vi "WPI_CANTalonSRX_RequestParameter.vi"(8 "error in (no error)":errorcluster, 10 "Parameter":T1=1 items=["Slot 0 - P"=1, "Slot 0 - I"=2, "Slot 0 - D"=3, "Slot 0 - F"=4, "Slot 0 - I Zone"=5, "Slot 0 - Ramp Rate"=6, "Slot 1 - P"=11, "Slot 1 - I"=12, "Slot 1 - D"=13, "Slot 1 - F"=14, "Slot 1 - I Zone"=15, "Slot 1 - Ramp Rate"=16, "Soft Limit - Forward"=21, "Soft Limit - Reverse"=22, "Soft Limit - Forward Enable"=23, "Soft Limit - Reverse Enable"=24, "On Boot - Brake Mode"=31, "On Boot - Limit Normally Closed - Forward"=32, "On Boot - Limit Normally Closed - Reverse"=33, "On Boot - Limit Disabled - Forward"=34, "On Boot - Limit Disabled - Reverse"=35, "Fault - Over Temp"=41, "Fault - Under Voltage"=42, "Fault - Forward Limit"=43, "Fault - Reverse Limit"=44, "Fault - Hardware Failure"=45, "Fault - Forward Soft Limit"=46, "Fault - Reverse Soft Limit"=47, "Sticky Fault - Over Temp"=48, "Sticky Fault - Under Voltage"=49, "Sticky Fault - Forward Limit"=50, "Sticky Fault - Reverse Limit"=51, "Sticky Fault - Forward Soft Limit"=52, "Sticky Fault - Reverse Soft Limit"=53, "Applied Throttle"=61, "Closed-Loop Error"=62, "Select Feedback Device"=63, "Reverse Closed-Loop Output"=64, "Mode Select"=65, "Profile Slot Select"=66, "Ramp Throttle"=67, "Reverse Feedback Sensor"=68, "Limit Switch Enabled"=69, "Limit Switch Closed - Forward"=70, "Limit Switch Closed - Reverse"=71, "Sensor Position"=73, "Sensor Velocity"=74, "Current"=75, "Brake is Enabled"=76, "Encoder Position"=77, "Encoder Velocity"=78, "Encoder Index Rise Events"=79, "Encoder A Pin State"=80, "Encoder B Pin State"=81, "Encoder Index Pin State"=82, "Analog In with Overflow"=83, "Analog In Velocity"=84, "Temperature"=85, "Battery Voltage"=86, "Reset Count"=87, "Reset Flags"=88, "Firmware Version"=89, "Settings Changed"=90, "Quad Filter Enable"=91, "Ignore Disable Broadcast"=92, "I Accumulator"=93, "Status 1 Frame Rate Ms"=94, "Status 2 Frame Rate Ms"=95, "Status 3 Frame Rate Ms"=96, "Status 4 Frame Rate Ms"=97, "Status 6 Frame Rate Ms"=98, "Status 7 Frame Rate Ms"=99, "Enable Index Pin Clear Position"=100, "Peak Positive Output"=104, "Nominal Positive Output"=105, "Peak Negative Output"=106, "Nominal Negative Output"=107, "Quad Index Pin Polarity"=108, "Status 8 Frame Rate Ms"=109, "Allow Position Overflow"=110, "Slot 0 - Allowable Closed-Loop Error"=111, "Number Potentiometer Turns"=112, "Encoder Codes Per Rev"=113, "Pulse Width Decoded Position"=114, "Analog Position"=115, "Voltage Compensation Rate (V/s)"=116, "Slot 1 - Allowable Closed-Loop Error"=117, "Motion Profile Has Underrun Err"=119, "Reserved 120"=120, "Legacy Control Mode"=121, "Motion Magic Acceleration"=122, "Motion Magic Cruise Velocity"=123, "Status 10 Frame Rate"=124, "Current Limit Threshold"=125], 11 "Device ID (0)":u8) -> (0 "error out":errorcluster, 3 "Device ID Out":u8)   [LabVIEW 2016]
uses:
  WPI_CANTalonSRX_Params.ctl
  WPI_CANTalonSRX_MessageIDs.ctl
  WPI_CANTalonSRX_GlobalOps.ctl
  WPI_CANTalonSRX_GlobalStatus.ctl
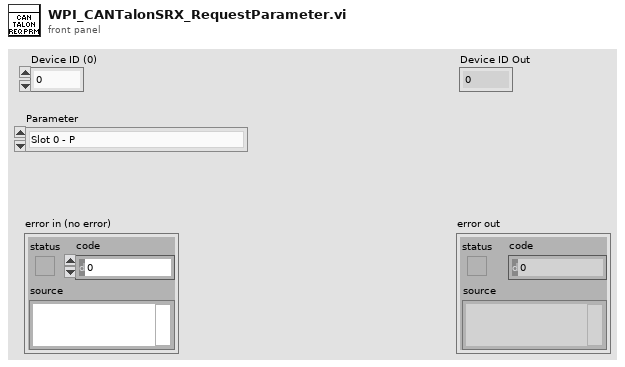
[diagram p1: front panel]
types:
  T1 = typedef "WPI_CANTalonSRX_Params.ctl" = u8
  T2 = typedef "WPI_CANTalonSRX_GlobalOps.ctl" = enum16{"Read For Send", "Write After Receive General", "Write After Receive Feedback", "Write After Receive Encoder", "Write After Receive Ain", "Write Error", "Get All", "Set Output", "Set Mode", "Set Master ID", "Set Brake Mode", "Set Reverse Feedback Sensor", "Set Reverse Closed Loop Output", "Set Override Limits", "Set Forward Limit Enabled", "Set Reverse Limit Enabled", "Set Feedback Select", "Set Profile Select", "Set Throttle Ramp Rate", "Disable", "Set Enc Codes Per Rev", "Set Num Pot Turns", "Set Control Frame Rate", "Enable Legacy Control", "Write After Receive Pulse Width", "Set Enable Frame Rate", "Write After Receive Motion Profile", "Set Motion Profile Flow Control", "Set Motion Profile Control Frame Rate", "Set Current Limit Enable"}
  T3 = typedef "WPI_CANTalonSRX_GlobalStatus.ctl" = cluster{"Applied Throttle":dbl, "Module Enabled":bool, "CAN Error":errorcluster, "Closed Loop Error":dbl, "Forward Limit Switch Closed":bool, "Reverse Limit Switch Closed":bool, "Sensor Position":dbl, "Sensor Velocity":dbl, "Current":dbl, "Sticky Fault - Over Temp":bool, "Sticky Fault - Under Voltage":bool, "Sticky Fault - Forward Limit":bool, "Sticky Fault - Reverse Limit":bool, "Sticky Fault - Forward Soft Limit":bool, "Sticky Fault - Reverse Soft Limit":bool, "Brake is Enabled":bool, "Encoder Position":dbl, "Encoder Velocity":dbl, "Encoder Index Count":dbl, "Encoder A Pin State":bool, "Encoder B Pin State":bool, "Encoder Index Pin State":bool, "Analog In":dbl, "Analog In Velocity":dbl, "Temperature (C)":dbl, "Battery Voltage":dbl, "Control 5 Is Supported":bool, "Current Profile Slot Select":dbl, "Pos Div 8":bool, "Vel Div 4":bool, "Pulse Width Position":i32, "Pulse Width Velocity":i32, "Pulse Width Rise To Rise (us)":i32, "Pulse Width Rise To Fall (us)":i32, "Mot Prof Active Is Under Run":bool, "Mot Prof Active Has Under Run":bool, "Mot Prof Active Is Last":bool, "Mot Prof Active Velocity Only":bool, "Mot Prof Active Is Valid":bool, "Mot Prof Buffer Is Full":bool, "Mot Prof Active Profile Slot Select":i32, "Mot Prof NextID":i32, "Mot Prof Count":i32, "Mot Prof Active Velocity":dbl, "Mot Prof Active Position":dbl, "Mot Prof Output Enable":i32}
  T4 = typedef "WPI_CANTalonSRX_MessageIDs.ctl" = u32
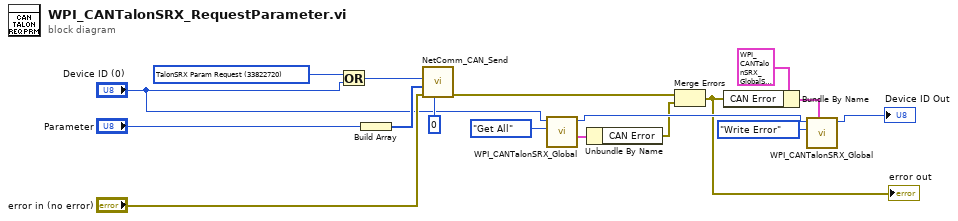
[diagram p0: block diagram]
diagram:
  w16 = T4 33822720 items=["TalonSRX Control General 10ms"=33816576, "TalonSRX Control Rates Slow"=33816640, "TalonSRX Control ClearFlags Slow"=33816704, "TalonSRX Status General 10ms"=33821696, "TalonSRX Status Feedback 20ms"=33821760, "TalonSRX Status Enc 100ms"=33821824, "TalonSRX Status AinTempVbat 100ms"=33821888, "TalonSRX Status Startup Once"=33821952, "TalonSRX Status Debug"=33822080, "TalonSRX Config SetGainsSlot0 A"=33823808, "TalonSRX Config SetGainsSlot0 B"=33823872, "TalonSRX Config SetGainsSlot1 A"=33823936, "TalonSRX Config SetGainsSlot1 B"=33824000, "TalonSRX Config SetSoftLimits"=33824064, "TalonSRX Config WebControl"=33824128, "TalonSRX Param Request"=33822720, "TalonSRX Param Response"=33822784, "TalonSRX Param Set"=33822848]
  n1 = Or(x=w16, y="Device ID (0)") -> (x .or. y?=w15:T4)
  n2 = Build Array("Parameter") -> (w17:T1[])
  n3 = call <vilib>:"NetComm_CAN_Send.vi"("Period (ms)"=0 ("milliseconds to wait"), "error in (no error)"="error in (no error)", "Data"=w17, "Message ID"=w15) -> ("error out"=w4:errorcluster)  [unwired: 7 in]
  n4 = call "WPI_CANTalonSRX_Global.vi"("Operation"=WPI_CANTalonSRX_GlobalOps."Get All", "Device ID (0)"="Device ID (0)") -> ("Get All"=w7:T3, "Device ID Out"=w5:u8)  [unwired: 7 in, 1 out]
  n5 = Unbundle By Name(w7) -> ("CAN Error"=w3:errorcluster)
  n6 = Merge Errors(w4, w3) -> (w1:errorcluster)
  "error out" <- w1
  n7 = Bundle By Name(cluster=T3 {"Applied Throttle"=0.0, "Module Enabled"=FALSE, "CAN Error"={"status"=FALSE, "code"=0, "source"=""}, "Closed Loop Error"=0.0, "Forward Limit Switch Closed"=FALSE, "Reverse Limit Switch Closed"=FALSE, "Sensor Position"=0.0, "Sensor Velocity"=0.0, "Current"=0.0, "Sticky Fault - Over Temp"=FALSE, "Sticky Fault - Under Voltage"=FALSE, "Sticky Fault - Forward Limit"=FALSE, "Sticky Fault - Reverse Limit"=FALSE, "Sticky Fault - Forward Soft Limit"=FALSE, "Sticky Fault - Reverse Soft Limit"=FALSE, "Brake is Enabled"=FALSE, "Encoder Position"=0.0, "Encoder Velocity"=0.0, "Encoder Index Count"=0.0, "Encoder A Pin State"=FALSE, "Encoder B Pin State"=FALSE, "Encoder Index Pin State"=FALSE, "Analog In"=0.0, "Analog In Velocity"=0.0, "Temperature (C)"=0.0, "Battery Voltage"=0.0, "Control 5 Is Supported"=FALSE, "Current Profile Slot Select"=0.0, "Pos Div 8"=FALSE, "Vel Div 4"=FALSE, "Pulse Width Position"=0, "Pulse Width Velocity"=0, "Pulse Width Rise To Rise (us)"=0, "Pulse Width Rise To Fall (us)"=0, "Mot Prof Active Is Under Run"=FALSE, "Mot Prof Active Has Under Run"=FALSE, "Mot Prof Active Is Last"=FALSE, "Mot Prof Active Velocity Only"=FALSE, "Mot Prof Active Is Valid"=FALSE, "Mot Prof Buffer Is Full"=FALSE, "Mot Prof Active Profile Slot Select"=0, "Mot Prof NextID"=0, "Mot Prof Count"=0, "Mot Prof Active Velocity"=0.0, "Mot Prof Active Position"=0.0, "Mot Prof Output Enable"=0} ("Write After Receive"), "CAN Error"=w1) -> (w11:T3)
  n8 = call "WPI_CANTalonSRX_Global.vi"("Write After Receive"=w11, "Operation"=WPI_CANTalonSRX_GlobalOps."Write Error", "Device ID (0)"=w5) -> ("Device ID Out"=→"Device ID Out":u8)  [unwired: 6 in, 2 out]
